vi "swerve_odometry.vi"(1 "input vector":T1, 3 "Delta Theta (deg)":dbl, 4 "Reset?":bool) -> (7 "Pose":dbl[](array[numeric]))   [LabVIEW 2020]
doc: "This VI calculates the field-centric delta odometry and velocity vectors for a single swerve module."
uses:
  <vilib>/Analysis/Matrix/Datatypes/RealMatrix.ctl
  <vilib>/Analysis/_algsub.llb/Vector Norm.vi
  <vilib>/Analysis/_algsub.llb/Real Vector Norm.vi
  <vilib>/Analysis/baseanly.llb/Outer Product.vi
  <vilib>/Analysis/baseanly.llb/Real Outer Product.vi
  <vilib>/robotics/Kinematics/Create Lie Group Matrix.vi
  <vilib>/Analysis/7linalg.llb/Create Special Matrix.vi
  <vilib>/Analysis/7linalg.llb/Create Special Real Matrix.vi
  <vilib>/Analysis/Matrix/Numeric/Multiply/Multiply - RM,R.vi
  <vilib>/Analysis/Matrix/Numeric/Multiply/Multiply - R,RM.vi
  <vilib>/Analysis/Matrix/Numeric/Add/Add.vi
  <vilib>/Analysis/Matrix/Numeric/Add/Add - RM,RM.vi
  <vilib>/Analysis/Matrix/Numeric/Conversions/Array To Matrix - RA2.vi
  <vilib>/Analysis/Matrix/Numeric/Multiply/Multiply - RM,RM.vi
  <vilib>/Analysis/Matrix/Numeric/Conversions/Matrix To Array - RM.vi
  <vilib>/robotics/Kinematics/NI_Kinematics.lvlib
  <vilib>/Analysis/Matrix/NI_Matrix.lvlib
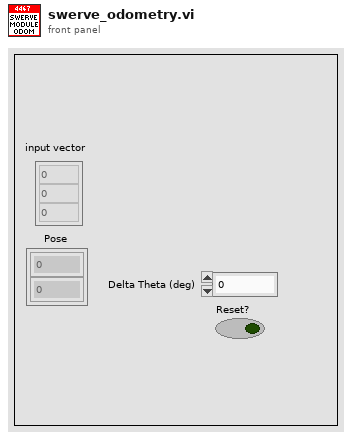
[diagram p1: front panel]
types:
  T1 = typedef "NI_Matrix.lvlib/RealMatrix.ctl" = dbl[][]
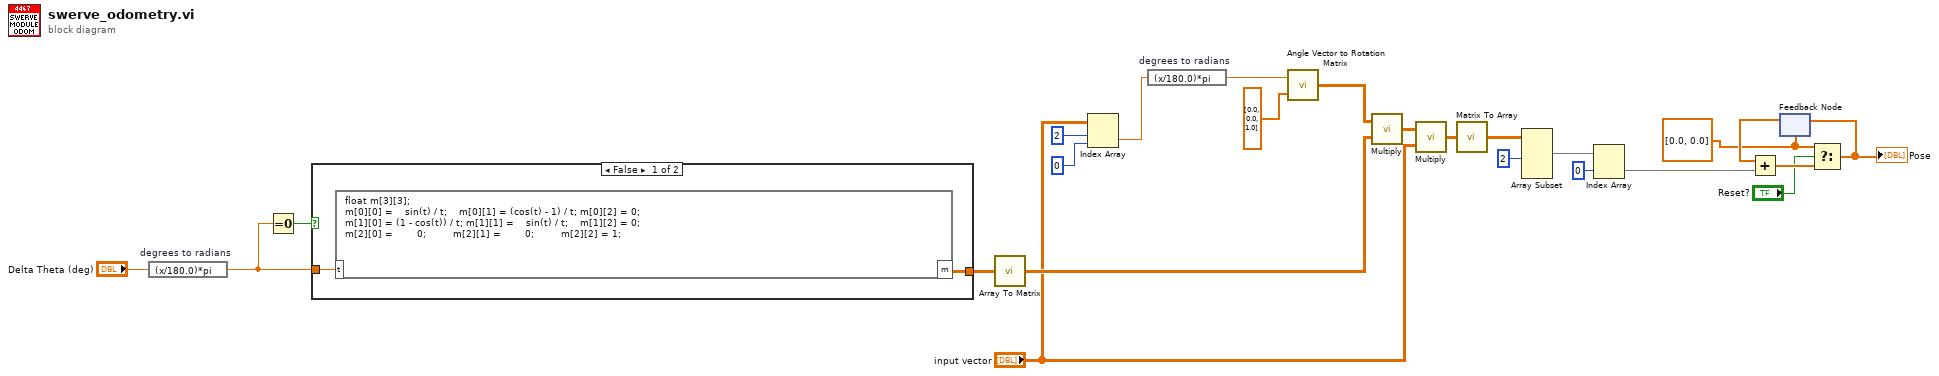
[diagram p0: block diagram]
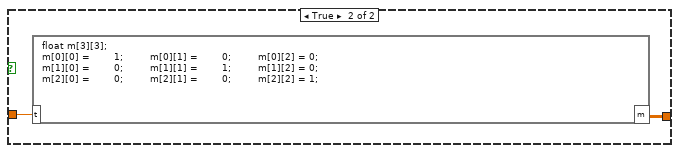
[diagram p2: hidden frame]
diagram:
  w1 = dbl[] [0.0, 0.0] ("t")
  n1 = expression code="(x/180.0)*pi" "degrees to radians"("Delta Theta (deg)") -> (w12:dbl)
  n2 = Equal To 0?(x=w12) -> (x = 0?=w13:bool)
  n3 = case shown="False" w13 {
    tunnel: w12 -> [w26 w28]
    tunnel: [w25 w27] -> w14
    frame False {
      n4 = formula code="float m[3][3];\nm[0][0] =    sin(t) / t;    m[0][1] = (cos(t) - 1) / t; m[0][2] = 0;\nm[1][0] = (1 - cos(t)) / t; m[1][1] =    sin(t) / t;    m[1][2] = 0;\nm[2][0] =        0;         m[2][1] =        0;         m[2][2] = 1;"("t"=w26) -> ("m"=w25:dbl[][])
    }
    frame True {
      n5 = formula code="float m[3][3];\nm[0][0] =        1;         m[0][1] =        0;         m[0][2] = 0;\nm[1][0] =        0;         m[1][1] =        1;         m[1][2] = 0;\nm[2][0] =        0;         m[2][1] =        0;         m[2][2] = 1;"("t"=w28) -> ("m"=w27:dbl[][])
    }
  }
  n6 = call-poly <vilib>:"Array To Matrix.vi"("Real 2D Array"=w14) -> ("Real Matrix"=w11:T1)
  n7 = Index Array(array="input vector", index (row)=2, index (col)=0) -> (element=w5:dbl)
  n8 = expression code="(x/180.0)*pi" "degrees to radians"(w5) -> (w21:dbl)
  n9 = call <vilib>:"Angle Vector to Rotation Matrix.vi"("vector"=dbl[] [0.0, 0.0, 1.0], "angle"=w21) -> ("rotation matrix"=w23:T1)
  n10 = call-poly <vilib>:"Multiply.vi"("Real Matrix B"=w11, "Real Matrix A"=w23) -> ("A * B"=w22:T1)
  n11 = call-poly <vilib>:"Multiply.vi"("Real Matrix B"="input vector", "Real Matrix A"=w22) -> ("A * B"=w16:T1)
  n12 = call-poly <vilib>:"Matrix To Array.vi"("Real Matrix"=w16) -> ("Real 2D Array"=w15:dbl[][])
  n13 = Array Subset(array=w15, length (row)=2 ("length")) -> (w19:dbl[][])  [unwired: 3 in]
  n14 = Index Array(array=w19, index (col)=0 ("disabled index (col)")) -> (element=w6:dbl[])  [unwired: 1 in]
  n15 = feedback #1(w1) -> (w8:dbl[])
  n16 = Add(x=w8, y=w6) -> (x+y=w9:dbl[])
  n17 = Select(t=w1, s="Reset?", f=w9) -> (s? t:f=w10:dbl[])
  "Pose" <- w10
  n18 = feedback-in #1(w10) -> ()
